vi "User ev LV2.vi"(0 "Stop":bool=TRUE, 11 "Error in":errorcluster, 13 "User Event Operator":T1) -> (4 "Stop":refnum<user-event>, 15 "Error out":errorcluster)   [LabVIEW 2020, in "I2C Controller.lvlib"]
uses:
  I2C Controller.lvlib
  Typedefs/User event operator.ctl
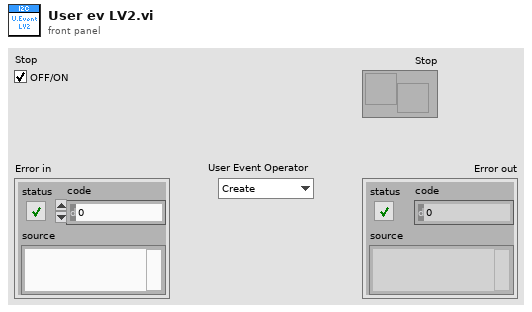
[diagram p1: front panel]
types:
  T1 = typedef "I2C Controller.lvlib/User event operator.ctl" = enum16{"Create", "Generate Stop", "Destroy"}
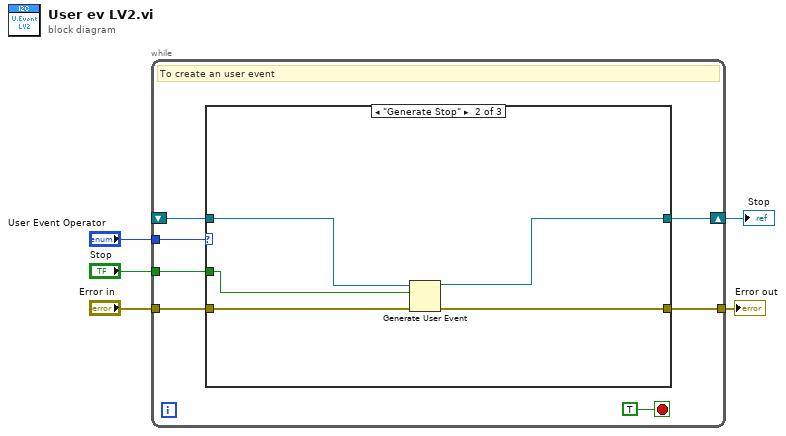
[diagram p0: block diagram]
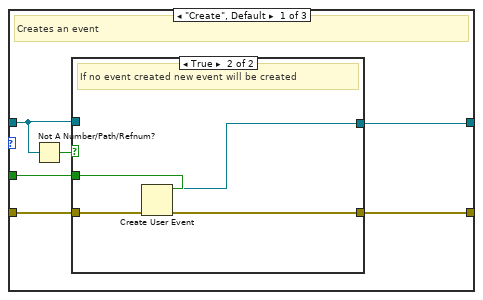
[diagram p2: hidden frame]
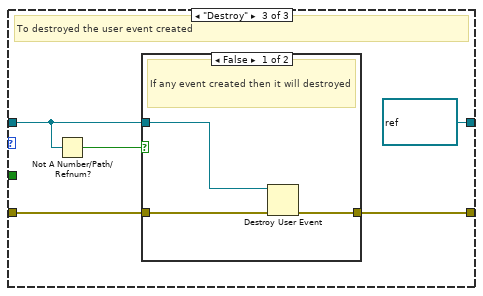
[diagram p4: hidden frame]
diagram:
  n1 = while {
    tunnel: "User Event Operator" -> [w12]
    tunnel: "Stop" -> [w11]
    tunnel: "Error in" -> [w10]
    shift-right: [w9] -> w1
    shift-left: _ -> [w8]
    tunnel: [w7] -> w2
    stop <- TRUE stop-if-true
    # "To create an user event"
    n2 = case shown="\"Generate Stop\"" w12 {
      tunnel: w11 -> [w15 w26 _]
      tunnel: w10 -> [w16 w29 w34]
      tunnel: [w14 w25 refnum<user-event> refnum ("Stop")] -> w9
      tunnel: w8 -> [w17 w27 w32]
      tunnel: [w13 w28 w33] -> w7
      frame "Create", Default {
        # "Creates an event"
        n3 = Not A Number/Path/Refnum?(number/path/refnum=w17) -> (NaN/Path/Refnum?=w18:bool)
        n4 = case shown="True" w18 {
          tunnel: w16 -> [w19 w24]
          tunnel: w15 -> [_ w23]
          tunnel: [w20 w22] -> w14
          tunnel: w17 -> [w20 _]
          tunnel: [w19 w21] -> w13
          frame False {
            # "If an event is created new event will not created again"
          }
          frame True {
            # "If no event created new event will be created"
            n5 = Create User Event(user event datatype=w23, error in=w24) -> (user event=w22:refnum<user-event>, error out=w21:errorcluster)
          }
        }
      }
      frame "Generate Stop" {
        n6 = Generate User Event(user event=w27, event data cluster=w26, error in=w29) -> (user event out=w25:refnum<user-event>, error out=w28:errorcluster)  [unwired: 1 in]
      }
      frame "Destroy" {
        # "To destroyed the user event created"
        n7 = Not A Number/Path/Refnum?(number/path/refnum=w32) -> (NaN/Path/Refnum?=w30:bool)
        n8 = case shown="False" w30 {
          tunnel: [w36 w38] -> w33
          tunnel: w34 -> [w37 w38]
          tunnel: w32 -> [w35 _]
          frame False {
            # "If any event created then it will destroyed"
            n9 = Destroy User Event(user event=w35, error in=w37) -> (error out=w36:errorcluster)
          }
          frame True {
            # "If no event created the nothing gets destroyed"
          }
        }
      }
    }
  }
  "Error out" <- w2
  "Stop" <- w1
